vi "IncrementNewHandleMutation.vi"(4 "SerializableData_v2.ctl":path, 6 "Mutate_v2_to_v3.vi":path, 7 "New BlueSerializableVersion":u16, 8 "error in (no error)":errorcluster, 9 "HandleVersionMutation.vi":path, 10 "Application":refnum<vi>, 11 "LVClassLibrary Ref":refnum<vi>) -> (0 "error out":errorcluster, 2 "Application":refnum<vi>, 3 "LVClassLibrary Ref":refnum<vi>)   [LabVIEW 2019, in "BlueSerializationScripts.lvlib"]
uses:
  BlueSerializationScripts.lvlib
  5fe2d410-0e28-46d4-8026-a22eea862cbf.vi
  d0df80ac-2923-4adc-816e-e88660028ae1.vi
  <vilib>/Utility/error.llb/Clear Errors.vi
  BlueSerialProviderGlobal.vi
  <vilib>/Utility/traverseref.llb/Traverse for GObjects.vi
  BlueUtilityScripts/RefIsOwner.vi
  BlueUtilityScripts/BlueUtilityScripts.lvlib
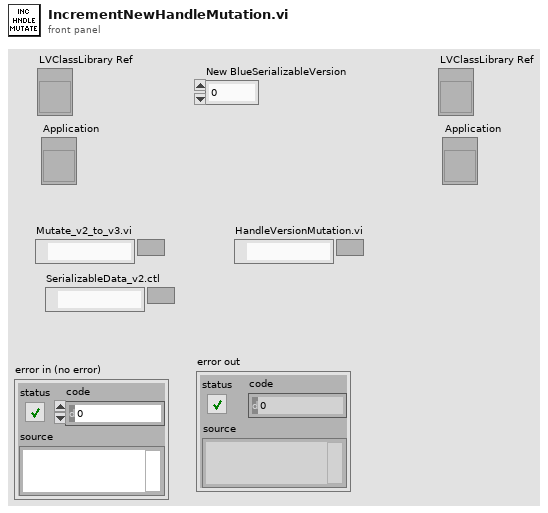
[diagram p1: front panel]
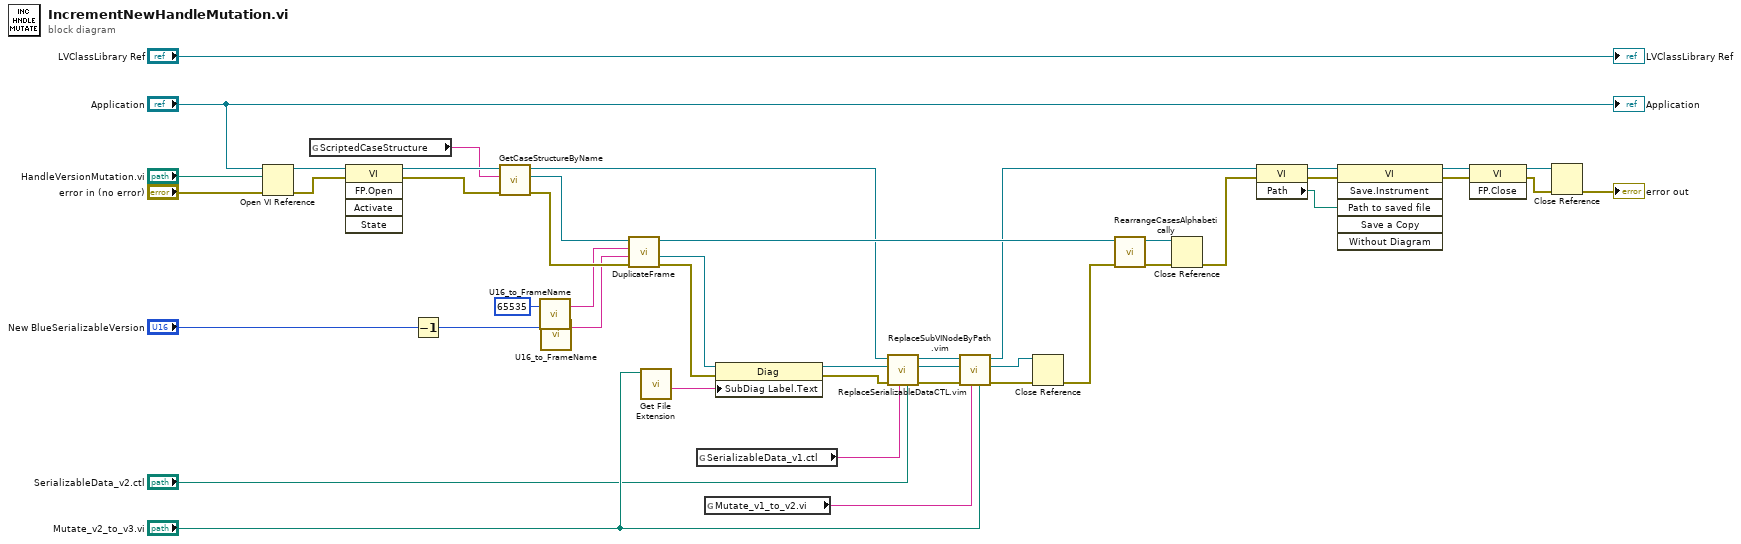
[diagram p0: block diagram]
diagram:
  n1 = Open VI Reference(application reference (local)="Application", vi path="HandleVersionMutation.vi", error in (no error)="error in (no error)") -> (vi reference=w40:refnum<vi>, error out=w39:errorcluster)  [unwired: 3 in]
  n2 = global read "BlueSerialProviderGlobal.vi" "ScriptedCaseStructure"() -> (w37:string)
  n3 = invoke class="VI" method="FP.Open"(reference=w40, error in=w39) -> (reference out=w38:refnum<vi>, error out=w36:errorcluster)  [unwired: 3 in, 3 out]
  n4 = Decrement(x="New BlueSerializableVersion") -> (x-1=w27:u16)
  n5 = call "GetCaseStructureByName.vi"("error in (no error)"=w36, "CaseStructureLabel.Text"=w37, "VI Refnum"=w38) -> ("error out"=w31:errorcluster, "CaseStructure Ref"=w35:refnum<vi>, "VI Refnum"=w5:refnum<vi>)  [unwired: 6 in]
  n6 = call "U16_to_FrameName.vi"("u16"=u16 65535) -> ("FrameName"=w29:string)  [unwired: 2 in]
  n7 = call "U16_to_FrameName.vi"("u16"=w27) -> ("FrameName"=w28:string)  [unwired: 2 in]
  n8 = call "DuplicateFrame.vi"("error in (no error)"=w31, "New FrameName"=w28, "FrameName to duplicate"=w29, "CaseStructure Ref"=w35) -> ("error out"=w25:errorcluster, "New Frame"=w26:refnum<vi>, "CaseStructure Ref"=w34:refnum<vi>)  [unwired: 5 in]
  n9 = call <vilib>:"Get File Extension.vi"("file"="Mutate_v2_to_v3.vi") -> ("filename without extension"=w14:string)  [unwired: 6 in, 4 out]
  n10 = global read "BlueSerialProviderGlobal.vi" "SerializableData_v1.ctl"() -> (w3:string)
  n11 = global read "BlueSerialProviderGlobal.vi" "Mutate_v1_to_v2.vi"() -> (w9:string)
  n12 = property class="Diag"(reference=w26, error in=w25, "SubDiag Label.Text"=w14) -> (reference out=w7:refnum<vi>, error out=w1:errorcluster)
  n13 = call "ReplaceSerializableDataCTL.vim"("CTL path"="SerializableData_v2.ctl", "TypedefPath Name"=w3, "error in (no error)"=w1, "Owner"=w7, "VI Refnum"=w5) -> ("error out"=w12:errorcluster, "dup Owner"=w6:refnum<vi>, "dup VI Refnum"=w4:refnum<vi>)  [unwired: 4 in]
  n14 = call "ReplaceSubVINodeByPath.vim"("SubVI  path"="Mutate_v2_to_v3.vi", "SubVI File Name"=w9, "error in (no error)"=w12, "Owner"=w6, "VI Refnum"=w4) -> ("error out"=w10:errorcluster, "dup Owner"=w11:refnum<vi>, "dup VI Refnum"=w13:refnum<vi>)  [unwired: 4 in]
  n15 = Close Reference(reference=w11, error in (no error)=w10) -> (error out=w24:errorcluster)
  n16 = call "RearrangeCasesAlphabetically.vi"("error in (no error)"=w24, "CaseStructure Ref"=w34) -> ("error out"=w32:errorcluster, "CaseStructure Ref"=w33:refnum<vi>)  [unwired: 8 in]
  n17 = Close Reference(reference=w33, error in (no error)=w32) -> (error out=w22:errorcluster)
  n18 = property class="VI"(reference=w13, error in=w22) -> (reference out=w23:refnum<vi>, error out=w20:errorcluster, "Path"=w21:path)
  n19 = invoke class="VI" method="Save.Instrument"(reference=w23, error in=w20, "Path to saved file"=w21) -> (reference out=w44:refnum<vi>, error out=w43:errorcluster)  [unwired: 3 in, 4 out]
  n20 = invoke class="VI" method="FP.Close"(reference=w44, error in=w43) -> (reference out=w42:refnum<vi>, error out=w41:errorcluster)  [unwired: 1 in, 1 out]
  n21 = Close Reference(reference=w42, error in (no error)=w41) -> (error out=→"error out":errorcluster)
  "LVClassLibrary Ref" <- "LVClassLibrary Ref"
  "Application" <- "Application"
